vi "Dump File Header Write.vi"(8 "error in":errorcluster, 10 "Raw Data Period":dbl=0.0001024, 11 "FPGA Refnum":T1) -> (0 "error out":errorcluster, 2 "concatenated string":string, 3 "Byte Stream File out":refnum<file>)   [LabVIEW 2022 SP3]
doc: "Author: Scott Hannahs <sth@magnet.fsu.edu>\nCopyright 2018 Florida State University, All rights reserved."
uses:
  RT Controls/FPGA SCH Digitizer Ref.ctl
  RT Host Globals.vi
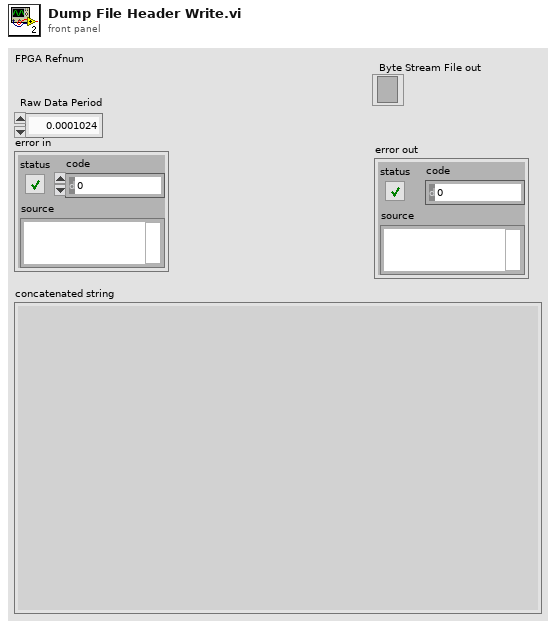
[diagram p1: front panel]
types:
  T1 = typedef "FPGA SCH Digitizer Ref.ctl" = refnum<k20>
  T2 = enum16{"open", "replace", "create", "open or create", "replace or create", "replace or create with confirmation"}
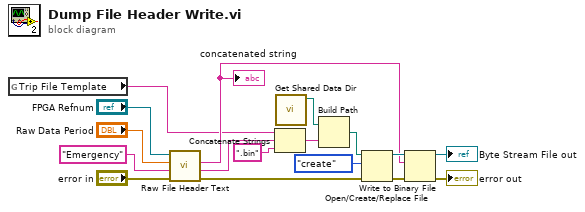
[diagram p0: block diagram]
diagram:
  n1 = global read "RT Host Globals.vi" "Trip File Template"() -> (w1:string)
  n2 = call "Raw File Header Text.vi"("error in (no error)"="error in", "Type"="Emergency", "Raw Data Period"="Raw Data Period", "FPGA Refnum out"="FPGA Refnum") -> ("error out"=w3:errorcluster, "Date String"=w6:string, "concatenated string"=w5:string)  [unwired: 5 in]
  "concatenated string" <- w5
  n3 = Concatenate Strings(w1, w6, ".bin" ("string")) -> (w15:string)
  n4 = call "Get Shared Data Dir.vi"() -> ("Data Directory Path"=w17:path)  [unwired: 2 in, 1 out]
  n5 = Build Path(base path=w17, name or relative path=w15) -> (appended path=w14:path)
  n6 = Open/Create/Replace File(file path (use dialog)=w14, error in=w3, operation (0:open)=T2."create") -> (refnum out=w11:refnum<file>, error out=w10:errorcluster)  [unwired: 3 in, 1 out]
  n7 = Write to Binary File(file (use dialog)=w11, data=w5, error in=w10) -> (refnum out=→"Byte Stream File out":refnum<file>, error out=→"error out":errorcluster)  [unwired: 3 in, 1 out]
